vi "_Remote Get Leybold Status.vi"(6 "UpdateError":bool, 7 "UpdatePump":bool, 8 "UpdateRunTime":bool, 9 "UpdatePower":bool, 10 "UpdateOthers":bool, 11 "UpdateConfig":bool) -> (0 "Run Time:":string[][](table)=[["Pump (hours)", ""], ["Days", ""], ["Number of Starts", ""], ["", ""], ["", ""], ["", ""], ["", ""], ["", ""]], 1 "Power:":string[][](table)=[["Voltage (V)", ""], ["Power (W)", ""], ["Current (A)", ""], ["Mean Current (A)", ""], ["Max Current (A)", ""], ["", ""], ["", ""], ["", ""]], 2 "OtherInfo":T1, 3 "Configuration:":string[][](table)=[["Pump Model", ""], ["Pump Serial Number", ""], ["Controller Model", ""], ["Controller Serial Number", ""], ["Electronics Model", ""], ["Electronic Serial Number", ""], ["Software Version", ""], ["Pump Parameter Set", ""]], 4 "Turbo OK":bool, 5 "Errors:":string[][](table)=[["0", ""], ["", ""], ["", ""], ["", ""], ["", ""], ["", ""], ["", ""], ["", ""]])   [LabVIEW 2012]
uses:
  Configuration/_Global Configuration.vi
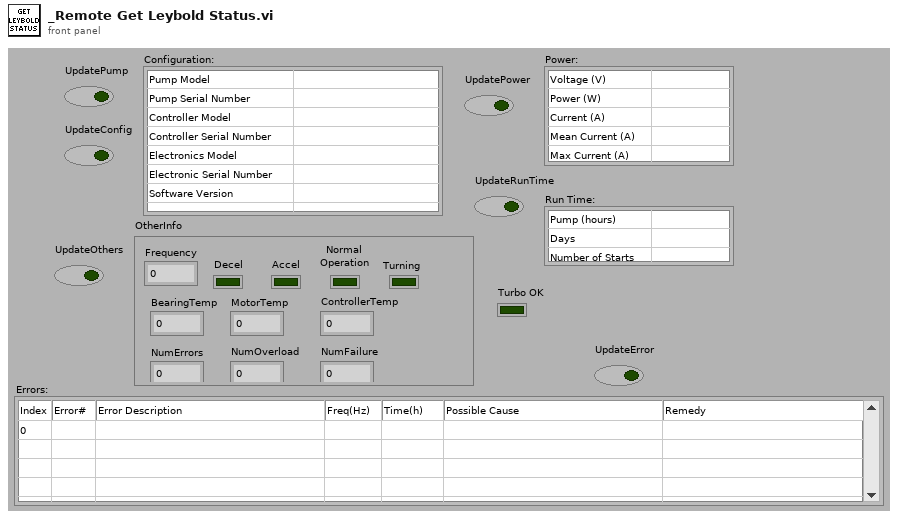
[diagram p1: front panel]
types:
  T1 = cluster{"Frequency":u16, "Decel":bool, "Accel":bool, "Normal \nOperation":bool, "Turning":bool, "BearingTemp":u32, "MotorTemp":u32, "ControllerTemp":u16, "PumpStatus":u16, "NumErrors":u32, "NumOverload":u32, "NumFailure":u32}
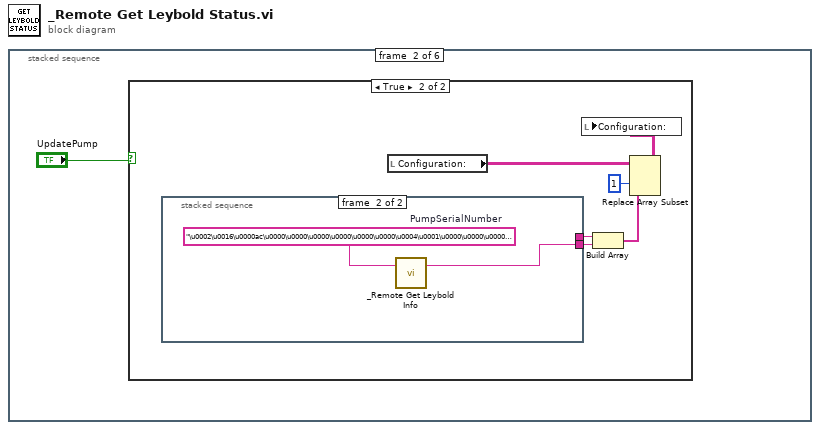
[diagram p0: block diagram]
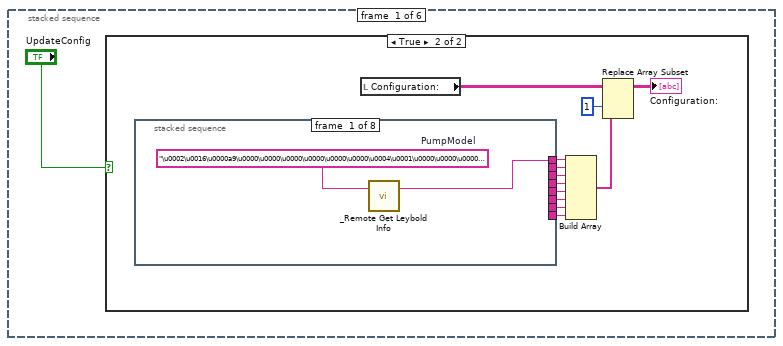
[diagram p2: hidden frame]
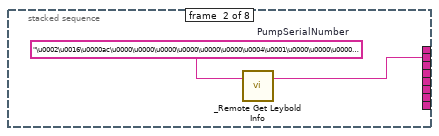
[diagram p4: hidden frame]
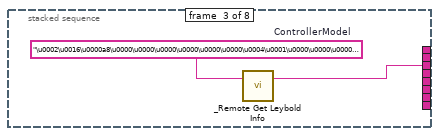
[diagram p5: hidden frame]
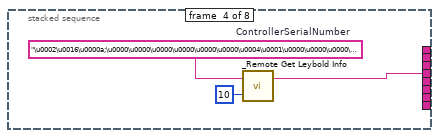
[diagram p6: hidden frame]
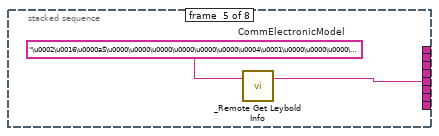
[diagram p7: hidden frame]
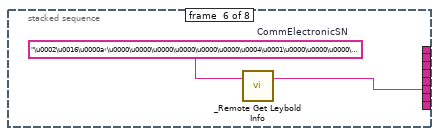
[diagram p8: hidden frame]
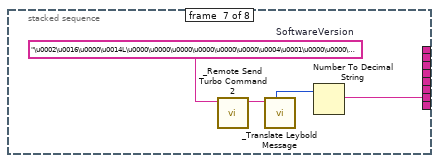
[diagram p9: hidden frame]
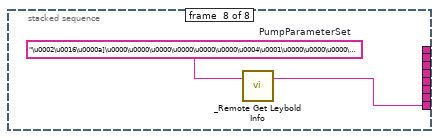
[diagram p10: hidden frame]
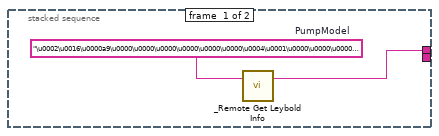
[diagram p12: hidden frame]
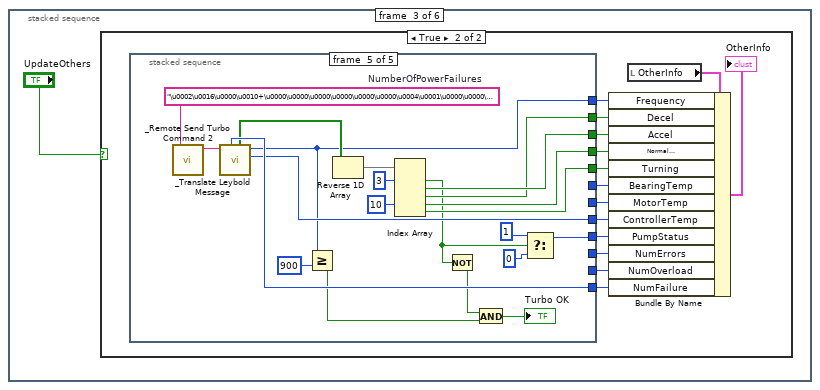
[diagram p13: hidden frame]
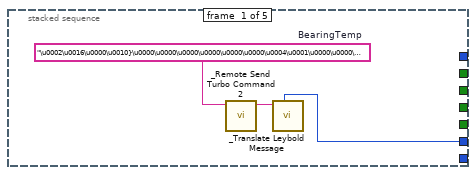
[diagram p15: hidden frame]
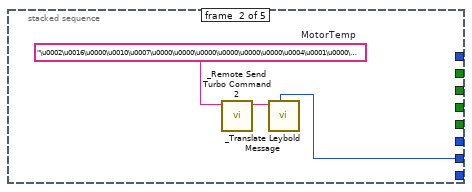
[diagram p16: hidden frame]
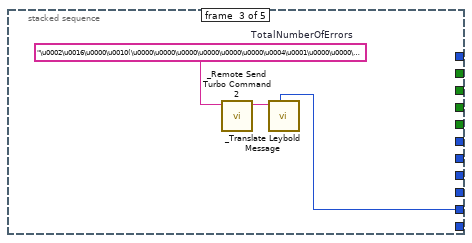
[diagram p17: hidden frame]
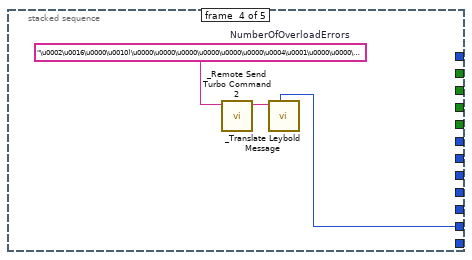
[diagram p18: hidden frame]
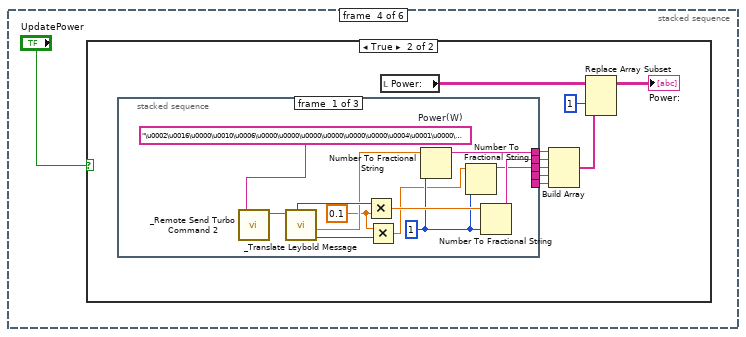
[diagram p19: hidden frame]
diagram:
  n1 = stacked-sequence {
    frame #0 {
      n2 = case shown="True" "UpdateConfig" {
        frame False {
        }
        frame True {
          n3 = stacked-sequence {
            tunnel: [w14 _ _ _ _ _ _ _] -> w11
            tunnel: [_ w16 _ _ _ _ _ _] -> w9
            tunnel: [_ _ w18 _ _ _ _ _] -> w8
            tunnel: [_ _ _ w21 _ _ _ _] -> w7
            tunnel: [_ _ _ _ w23 _ _ _] -> w6
            tunnel: [_ _ _ _ _ w25 _ _] -> w5
            tunnel: [_ _ _ _ _ _ _ w31] -> w4
            tunnel: [_ _ _ _ _ _ w27 _] -> w3
            frame #0 {
              w15 = "\u0002\u0016\u0000a9\u0000\u0000\u0000\u0000\u0000\u0000\u0004\u0001\u0000\u0000\u0000\u0000\u0000\u0000\u0000\u0000\u0000\u0000I"  # PumpModel
              n4 = call "_Remote Get Leybold Info.vi"("TemplateTelegram"=w15) -> ("Reply"=w14:string)  [unwired: 2 in]
            }
            frame #1 {
              w17 = "\u0002\u0016\u0000ac\u0000\u0000\u0000\u0000\u0000\u0000\u0004\u0001\u0000\u0000\u0000\u0000\u0000\u0000\u0000\u0000\u0000\u0000\u0013"  # PumpSerialNumber
              n5 = call "_Remote Get Leybold Info.vi"("TemplateTelegram"=w17) -> ("Reply"=w16:string)  [unwired: 2 in]
            }
            frame #2 {
              w19 = "\u0002\u0016\u0000a8\u0000\u0000\u0000\u0000\u0000\u0000\u0004\u0001\u0000\u0000\u0000\u0000\u0000\u0000\u0000\u0000\u0000\u0000H"  # ControllerModel
              n6 = call "_Remote Get Leybold Info.vi"("TemplateTelegram"=w19) -> ("Reply"=w18:string)  [unwired: 2 in]
            }
            frame #3 {
              w22 = "\u0002\u0016\u0000a;\u0000\u0000\u0000\u0000\u0000\u0000\u0004\u0001\u0000\u0000\u0000\u0000\u0000\u0000\u0000\u0000\u0000\u0000K"  # ControllerSerialNumber
              n7 = call "_Remote Get Leybold Info.vi"("#Index(18)"=u8 10, "TemplateTelegram"=w22) -> ("Reply"=w21:string)  [unwired: 1 in]
            }
            frame #4 {
              w24 = "\u0002\u0016\u0000aŠ\u0000\u0000\u0000\u0000\u0000\u0000\u0004\u0001\u0000\u0000\u0000\u0000\u0000\u0000\u0000\u0000\u0000\u0000ú"  # CommElectronicModel
              n8 = call "_Remote Get Leybold Info.vi"("TemplateTelegram"=w24) -> ("Reply"=w23:string)  [unwired: 2 in]
            }
            frame #5 {
              w26 = "\u0002\u0016\u0000a‹\u0000\u0000\u0000\u0000\u0000\u0000\u0004\u0001\u0000\u0000\u0000\u0000\u0000\u0000\u0000\u0000\u0000\u0000û"  # CommElectronicSN
              n9 = call "_Remote Get Leybold Info.vi"("TemplateTelegram"=w26) -> ("Reply"=w25:string)  [unwired: 2 in]
            }
            frame #6 {
              w29 = "\u0002\u0016\u0000\u0014L\u0000\u0000\u0000\u0000\u0000\u0000\u0004\u0001\u0000\u0000\u0000\u0000\u0000\u0000\u0000\u0000\u0000\u0000I"  # SoftwareVersion
              n10 = call "_Remote Send Turbo Command 2.vi"("Telegram"=w29) -> ("Raw Reply"=w30:string)  [unwired: 5 in, 1 out]
              n11 = call "_Translate Leybold Message.vi"("LeyboldMessage"=w30) -> ("Parameter"=w28:u32)  [unwired: 3 in, 7 out]
              n12 = Number To Decimal String(number=w28) -> (decimal integer string=w27:string)  [unwired: 1 in]
            }
            frame #7 {
              w32 = "\u0002\u0016\u0000a]\u0000\u0000\u0000\u0000\u0000\u0000\u0004\u0001\u0000\u0000\u0000\u0000\u0000\u0000\u0000\u0000\u0000\u0000-"  # PumpParameterSet
              n13 = call "_Remote Get Leybold Info.vi"("TemplateTelegram"=w32) -> ("Reply"=w31:string)  [unwired: 2 in]
            }
          }
          n14 = local read "Configuration:"() -> (w13:string[][])
          n15 = Build Array(w11, w9, w8, w7, w6, w5, w3, w4) -> (w10:string[])
          n16 = Replace Array Subset(array=w13, new element=w10, index (col)=1 ("disabled index (col)")) -> (→"Configuration:":string[][])  [unwired: 1 in]
        }
      }
    }
    frame #1 {
      n17 = case shown="True" "UpdatePump" {
        frame False {
        }
        frame True {
          n18 = stacked-sequence {
            tunnel: [w40 _] -> w37
            tunnel: [_ w42] -> w35
            frame #0 {
              w41 = "\u0002\u0016\u0000a9\u0000\u0000\u0000\u0000\u0000\u0000\u0004\u0001\u0000\u0000\u0000\u0000\u0000\u0000\u0000\u0000\u0000\u0000I"  # PumpModel
              n19 = call "_Remote Get Leybold Info.vi"("TemplateTelegram"=w41) -> ("Reply"=w40:string)  [unwired: 2 in]
            }
            frame #1 {
              w43 = "\u0002\u0016\u0000ac\u0000\u0000\u0000\u0000\u0000\u0000\u0004\u0001\u0000\u0000\u0000\u0000\u0000\u0000\u0000\u0000\u0000\u0000\u0013"  # PumpSerialNumber
              n20 = call "_Remote Get Leybold Info.vi"("TemplateTelegram"=w43) -> ("Reply"=w42:string)  [unwired: 2 in]
            }
          }
          n21 = local read "Configuration:"() -> (w39:string[][])
          n22 = Build Array(w37, w35) -> (w36:string[])
          n23 = Replace Array Subset(array=w39, new element=w36, index (col)=1 ("disabled index (col)")) -> (w34:string[][])  [unwired: 1 in]
          n24 = local write "Configuration:"(w34) -> ()
        }
      }
    }
    frame #2 {
      n25 = case shown="True" "UpdateOthers" {
        frame False {
        }
        frame True {
          n26 = stacked-sequence {
            tunnel: [w59 _ _ _ _] -> w56
            tunnel: [_ w62 _ _ _] -> w55
            tunnel: [_ _ _ _ w88] -> w54
            tunnel: [_ _ w65 _ _] -> w53
            tunnel: [_ _ _ w68 _] -> w52
            tunnel: [_ _ _ _ w89] -> w51
            tunnel: [_ _ _ _ w75] -> w50
            tunnel: [_ _ _ _ w83] -> w49
            tunnel: [_ _ _ _ w82] -> w48
            tunnel: [_ _ _ _ w81] -> w47
            tunnel: [_ _ _ _ w80] -> w46
            tunnel: [_ _ _ _ w79] -> w45
            frame #0 {
              w60 = "\u0002\u0016\u0000\u0010}\u0000\u0000\u0000\u0000\u0000\u0000\u0004\u0001\u0000\u0000\u0000\u0000\u0000\u0000\u0000\u0000\u0000\u0000|"  # BearingTemp
              n27 = call "_Remote Send Turbo Command 2.vi"("Telegram"=w60) -> ("Raw Reply"=w61:string)  [unwired: 5 in, 1 out]
              n28 = call "_Translate Leybold Message.vi"("LeyboldMessage"=w61) -> ("Parameter"=w59:u32)  [unwired: 3 in, 7 out]
            }
            frame #1 {
              w63 = "\u0002\u0016\u0000\u0010\u0007\u0000\u0000\u0000\u0000\u0000\u0000\u0004\u0001\u0000\u0000\u0000\u0000\u0000\u0000\u0000\u0000\u0000\u0000\u0006"  # MotorTemp
              n29 = call "_Remote Send Turbo Command 2.vi"("Telegram"=w63) -> ("Raw Reply"=w64:string)  [unwired: 5 in, 1 out]
              n30 = call "_Translate Leybold Message.vi"("LeyboldMessage"=w64) -> ("Parameter"=w62:u32)  [unwired: 3 in, 7 out]
            }
            frame #2 {
              w66 = "\u0002\u0016\u0000\u0010(\u0000\u0000\u0000\u0000\u0000\u0000\u0004\u0001\u0000\u0000\u0000\u0000\u0000\u0000\u0000\u0000\u0000\u0000)"  # TotalNumberOfErrors
              n31 = call "_Remote Send Turbo Command 2.vi"("Telegram"=w66) -> ("Raw Reply"=w67:string)  [unwired: 5 in, 1 out]
              n32 = call "_Translate Leybold Message.vi"("LeyboldMessage"=w67) -> ("Parameter"=w65:u32)  [unwired: 3 in, 7 out]
            }
            frame #3 {
              w69 = "\u0002\u0016\u0000\u0010)\u0000\u0000\u0000\u0000\u0000\u0000\u0004\u0001\u0000\u0000\u0000\u0000\u0000\u0000\u0000\u0000\u0000\u0000("  # NumberOfOverloadErrors
              n33 = call "_Remote Send Turbo Command 2.vi"("Telegram"=w69) -> ("Raw Reply"=w70:string)  [unwired: 5 in, 1 out]
              n34 = call "_Translate Leybold Message.vi"("LeyboldMessage"=w70) -> ("Parameter"=w68:u32)  [unwired: 3 in, 7 out]
            }
            frame #4 {
              w90 = "\u0002\u0016\u0000\u0010+\u0000\u0000\u0000\u0000\u0000\u0000\u0004\u0001\u0000\u0000\u0000\u0000\u0000\u0000\u0000\u0000\u0000\u0000*"  # NumberOfPowerFailures
              n35 = call "_Remote Send Turbo Command 2.vi"("Telegram"=w90) -> ("Raw Reply"=w91:string)  [unwired: 5 in, 1 out]
              n36 = call "_Translate Leybold Message.vi"("LeyboldMessage"=w91) -> ("Temperature"=w88:u16, "Frequency"=w75:u16, "Pump Status"=w87:bool[], "Parameter"=w89:u32)  [unwired: 3 in, 4 out]
              n37 = Greater Or Equal?(x=w75, y=u16 900) -> (x >= y?=w72:bool)
              n38 = Reverse 1D Array(array=w87) -> (reversed array=w86:bool[])
              n39 = Index Array(array=w86, index #1=3 ("index"), index #4=10 ("index")) -> (element #1=w74:bool, element #2=w83:bool, element #3=w82:bool, element #4=w81:bool, element #5=w80:bool)  [unwired: 3 in]
              n40 = Not(x=w74) -> (.not. x?=w73:bool)
              n41 = And(x=w73, y=w72) -> (x .and. y?=→"Turbo OK":bool)
              n42 = Select(t=u16 1 ("PumpStatus"), s=w74, f=u16 0) -> (s? t:f=w79:u16)
            }
          }
          n43 = local read "OtherInfo"() -> (w58:T1)
          n44 = Bundle By Name(cluster=w58, "Frequency"=w50, "Decel"=w48, "Accel"=w49, "Normal \nOperation"=w47, "Turning"=w46, "BearingTemp"=w56, "MotorTemp"=w55, "ControllerTemp"=w54, "PumpStatus"=w45, "NumErrors"=w53, "NumOverload"=w52, "NumFailure"=w51) -> (→"OtherInfo":T1)
        }
      }
    }
    frame #3 {
      n45 = case shown="True" "UpdatePower" {
        frame False {
        }
        frame True {
          n46 = stacked-sequence {
            tunnel: [w107 _ _] -> w98
            tunnel: [w109 _ _] -> w97
            tunnel: [w103 _ _] -> w96
            tunnel: [_ w114 _] -> w95
            tunnel: [_ _ w121] -> w94
            frame #0 {
              w105 = i16 1 ("precision (6)")
              w102 = 0.1 ("y")
              w112 = "\u0002\u0016\u0000\u0010\u0006\u0000\u0000\u0000\u0000\u0000\u0000\u0004\u0001\u0000\u0000\u0000\u0000\u0000\u0000\u0000\u0000\u0000\u0000\u0007"  # Power(W)
              n47 = call "_Remote Send Turbo Command 2.vi"("Telegram"=w112) -> ("Raw Reply"=w113:string)  [unwired: 5 in, 1 out]
              n48 = call "_Translate Leybold Message.vi"("LeyboldMessage"=w113) -> ("Voltage"=w106:u16, "Current"=w108:dbl, "Parameter"=w111:u32)  [unwired: 3 in, 5 out]
              n49 = Multiply(x=w111, y=w102) -> (x*y=w110:dbl)
              n50 = Multiply(x=w102, y=w106) -> (x*y=w104:dbl)
              n51 = Number To Fractional String(number=w108, precision (6)=w105) -> (F-format string=w107:string)  [unwired: 2 in]
              n52 = Number To Fractional String(number=w104, precision (6)=w105) -> (F-format string=w103:string)  [unwired: 2 in]
              n53 = Number To Fractional String(number=w110, precision (6)=w105) -> (F-format string=w109:string)  [unwired: 2 in]
            }
            frame #1 {
              w119 = "\u0002\u0016\u0000\u0010\u0000\u0000\u0000\u0000\u0000\u0000\u0004\u0001\u0000\u0000\u0000\u0000\u0000\u0000\u0000\u0000\u0000\u0000"  # MeanCurrent
              n54 = call "_Remote Send Turbo Command 2.vi"("Telegram"=w119) -> ("Raw Reply"=w120:string)  [unwired: 5 in, 1 out]
              n55 = call "_Translate Leybold Message.vi"("LeyboldMessage"=w120) -> ("Parameter"=w115:u32)  [unwired: 3 in, 7 out]
              n56 = Multiply(x=w115, y=0.1) -> (x*y=w117:dbl)
              n57 = Number To Fractional String(number=w117, precision (6)=i16 1) -> (F-format string=w114:string)  [unwired: 2 in]
            }
            frame #2 {
              w126 = "\u0002\u0016\u0000\u0010¹\u0000\u0000\u0000\u0000\u0000\u0000\u0004\u0001\u0000\u0000\u0000\u0000\u0000\u0000\u0000\u0000\u0000\u0000¸"  # MaxCurrent
              n58 = call "_Remote Send Turbo Command 2.vi"("Telegram"=w126) -> ("Raw Reply"=w127:string)  [unwired: 5 in, 1 out]
              n59 = call "_Translate Leybold Message.vi"("LeyboldMessage"=w127) -> ("Parameter"=w122:u32)  [unwired: 3 in, 7 out]
              n60 = Multiply(x=w122, y=0.1) -> (x*y=w124:dbl)
              n61 = Number To Fractional String(number=w124, precision (6)=i16 1) -> (F-format string=w121:string)  [unwired: 2 in]
            }
          }
          n62 = local read "Power:"() -> (w101:string[][])
          n63 = Build Array(w98, w97, w96, w95, w94) -> (w93:string[])
          n64 = Replace Array Subset(array=w101, new element=w93, index (col)=1 ("disabled index (col)")) -> (→"Power:":string[][])  [unwired: 1 in]
        }
      }
    }
    frame #4 {
      n65 = case shown="True" "UpdateRunTime" {
        frame False {
        }
        frame True {
          n66 = stacked-sequence {
            tunnel: [w143 _] -> w132
            tunnel: [w136 _] -> w131
            tunnel: [_ w147] -> w130
            frame #0 {
              w145 = "\u0002\u0016\u0000\u0010¸\u0000\u0000\u0000\u0000\u0000\u0000\u0004\u0001\u0000\u0000\u0000\u0000\u0000\u0000\u0000\u0000\u0000\u0000¹"  # PumpHours
              n67 = call "_Remote Send Turbo Command 2.vi"("Telegram"=w145) -> ("Raw Reply"=w146:string)  [unwired: 5 in, 1 out]
              n68 = call "_Translate Leybold Message.vi"("LeyboldMessage"=w146) -> ("Parameter"=w144:u32)  [unwired: 3 in, 7 out]
              n69 = Multiply(x=w144, y=0.01) -> (x*y=w140:dbl)
              n70 = Divide(x=w140, y=24.0) -> (x/y=w137:dbl)
              n71 = Number To Fractional String(number=w140, precision (6)=i16 2) -> (F-format string=w143:string)  [unwired: 2 in]
              n72 = Number To Fractional String(number=w137, precision (6)=i16 4) -> (F-format string=w136:string)  [unwired: 2 in]
            }
            frame #1 {
              w149 = "\u0002\u0016\u0000\u0010&\u0000\u0000\u0000\u0000\u0000\u0000\u0004\u0001\u0000\u0000\u0000\u0000\u0000\u0000\u0000\u0000\u0000\u0000'"  # NumberOfStarts
              n73 = call "_Remote Send Turbo Command 2.vi"("Telegram"=w149) -> ("Raw Reply"=w150:string)  [unwired: 5 in, 1 out]
              n74 = call "_Translate Leybold Message.vi"("LeyboldMessage"=w150) -> ("Parameter"=w148:u32)  [unwired: 3 in, 7 out]
              n75 = Number To Decimal String(number=w148) -> (decimal integer string=w147:string)  [unwired: 1 in]
            }
          }
          n76 = local read "Run Time:"() -> (w135:string[][])
          n77 = Build Array(w132, w131, w130) -> (w129:string[])
          n78 = Replace Array Subset(array=w135, new element=w129, index (col)=1 ("disabled index (col)")) -> (→"Run Time:":string[][])  [unwired: 1 in]
        }
      }
    }
    frame #5 {
      n79 = case shown="True" "UpdateError" {
        frame False {
        }
        frame True {
          n80 = global read "_Global Configuration.vi" "Advanced"() -> (w157:bool)
          n81 = local read "OtherInfo"() -> (w156:T1)
          n82 = Unbundle By Name(w156) -> ("NumErrors"=w154:u32)
          n83 = Select(t=w154, s=w157, f=u32 1) -> (s? t:f=w155:u32)
          n84 = for {
            N: w155 -> [_]
            tunnel: [w158] -> w152 mode=indexing
            i -> [w159]
            n85 = call "_Remote Get Leybold Error.vi"("ErrorIndex (0)"=w159) -> ("Reply"=w158:string[])  [unwired: 1 in, 1 out]
          }
          "Errors:" <- w152
        }
      }
    }
  }
